vi "RX-SIM-BPCS-UDP.vi"() -> ()   [LabVIEW 2018]
uses:
  <vilib>/Platform/TimedLoop/XDataNode/timing_clust.ctl
  <vilib>/Platform/TimedLoop/XDataNode/nitl_modes.ctl
  <vilib>/Platform/TimedLoop/XDataNode/wakeup.ctl
  Modbus/ControllersHost/BPCS Global Variables.vi
  <vilib>/Platform/TimedLoop/XDataNode/XDataNode.xnode
  <vilib>/Platform/TimedLoop/XDataNode/XDNodeRunTimeDep.lvlib
panel:
  in  "Stop":bool
  out "SIM-BPCS-RX-ARRAY":dbl[](array[numeric])
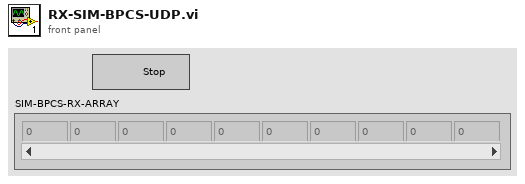
[diagram p1: front panel]
types:
  T1 = typedef "XDNodeRunTimeDep.lvlib/timing_clust.ctl" = cluster{"Expected End [f-1]":u64, "Actual End [f-1]":u64, "Finished Late? [f-1]":bool, "Expected End [i-1]":u64, "Actual End [i-1]":u64, "Finished Late? [i-1]":bool, "Expected Start [i]":u64, "Actual Start [i]":u64, "Expected Start [f]":u64, "Actual Start [f]":u64, "Source Name":string, "Structure Name":string, "Period":i64, "Deadline":i64, "Offset":i64, "Start":i64, "Priority":i32, "Timeout":i32, "Mode":T2, "Wakeup Reason":T3, "Error":errorcluster, "Source Type":string, "Secondary Source Type":string, "Global End Time":u64, "Global Start Time":u64, "Frame Duration":u64, "Iteration Duration":u64, "Assigned CPU":i32, "I/O Scan Engine Mode":u32}
  T2 = typedef "XDNodeRunTimeDep.lvlib/nitl_modes.ctl" = enum32{"No Change", "Process missed periods, maintain original phase", "Discard missed periods, maintain original phase", "Process missed periods, ignore original phase", "Discard missed periods, ignore original phase"}
  T3 = typedef "XDNodeRunTimeDep.lvlib/wakeup.ctl" = enum32{"Normal", "Aborted", "Asynchronous wakeup", "Timing source error", "Timed loop error", "Timeout"}
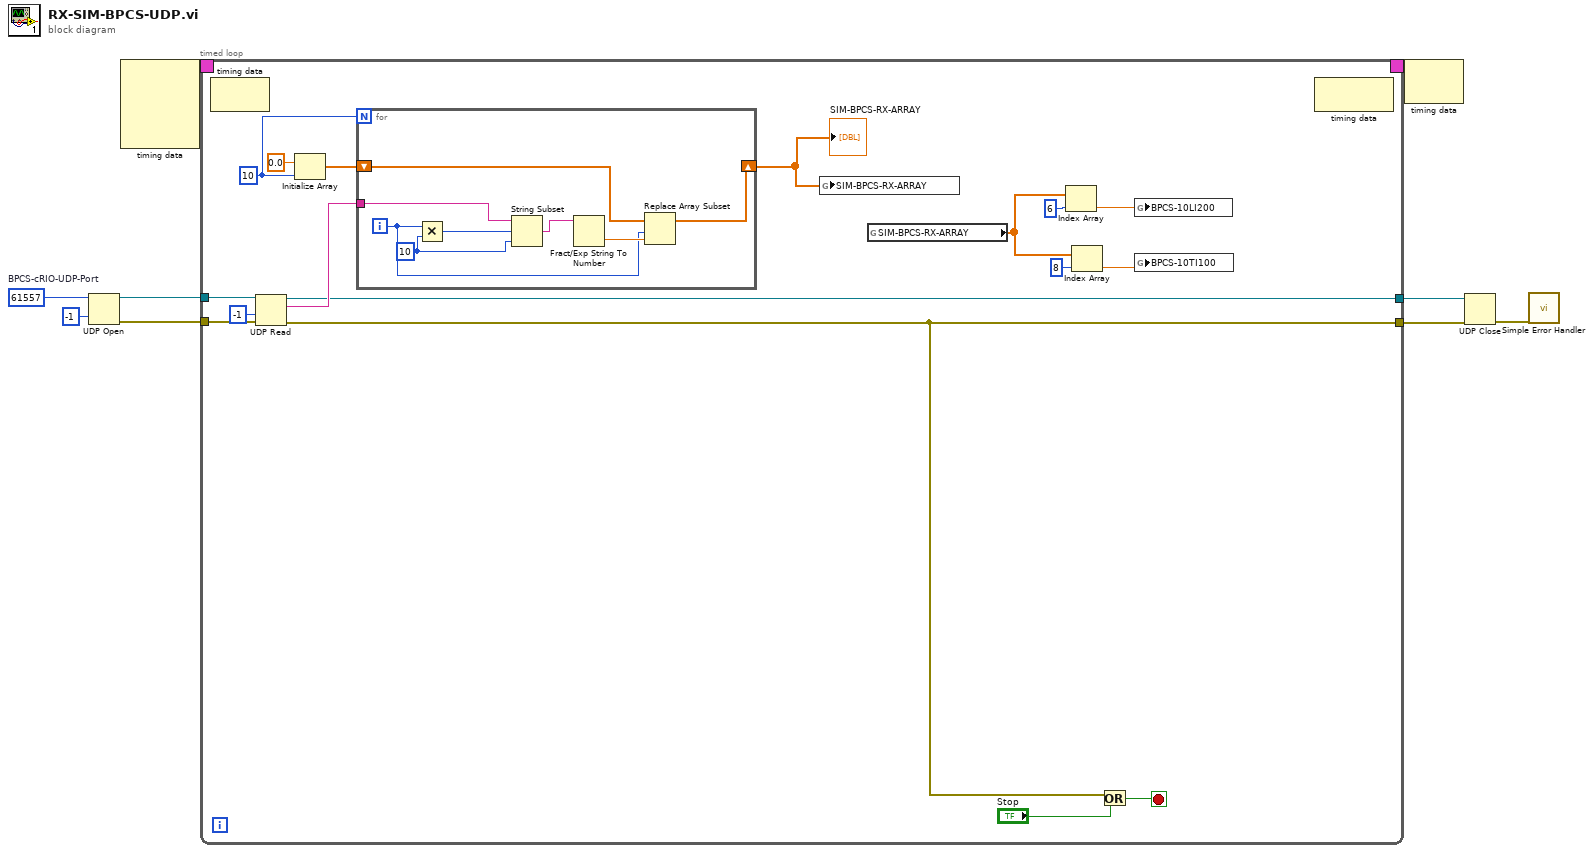
[diagram p0: block diagram]
diagram:
  w7 = u16 61557  # BPCS-cRIO-UDP-Port
  n1 = UDP Open(9:-1 ("timeout ms (25000)"), 11:w7) -> (port=w6:refnum<k16>, 0:w5:errorcluster)  [unwired: 3 in, 1 out]
  n2 = node-c288() -> (w9:T1)  [unwired: 4 in]
  n3 = timed-loop {
    timing: w9 -> [_]
    timing-out: [_] -> w8
    tunnel: w6 -> [w24]
    tunnel: w5 -> [w23]
    tunnel: [w21] -> w3
    tunnel: [w15] -> w1
    stop <- w25 stop-if-true
    w18 = 10 ("dimension size")
    n4 = node-c288() -> ()  [unwired: 1 in, 1 out]
    n5 = UDP Read(connection ID=w24, timeout ms (25000)=-1, 8:w23) -> (data out=w22:string, error out=w15:errorcluster, 3:w21:refnum<k16>)  [unwired: 3 out]
    n6 = Initialize Array(0.0 ("element"), w18) -> (w19:dbl[])
    n7 = for {
      N: w18 -> [_]
      tunnel: w22 -> [w33]
      shift-right: [w29] -> w16
      shift-left: w19 -> [w28]
      i -> [w30]
      w27 = 10 ("y")
      n8 = Multiply(x=w30, y=w27) -> (x*y=w32:i32)
      n9 = String Subset(string=w33, offset (0)=w32, length (rest)=w27) -> (substring=w34:string)
      n10 = Fract/Exp String To Number(string=w34) -> (number=w31:dbl)  [unwired: 3 in, 1 out]
      n11 = Replace Array Subset(array=w28, new element=w31, index=w30) -> (w29:dbl[])
    }
    "SIM-BPCS-RX-ARRAY" <- w16
    n12 = global write "BPCS Global Variables.vi" "SIM-BPCS-RX-ARRAY"(w16) -> ()
    n13 = global read "BPCS Global Variables.vi" "SIM-BPCS-RX-ARRAY"() -> (w12:dbl[])
    n14 = Index Array(array=w12, index=6) -> (element=w11:dbl)
    n15 = Index Array(array=w12, index=8) -> (element=w10:dbl)
    n16 = Or(x=w15, y="Stop") -> (x .or. y?=w25:bool)
    n17 = global write "BPCS Global Variables.vi" "BPCS-10LI200"(w11) -> ()
    n18 = global write "BPCS Global Variables.vi" "BPCS-10TI100"(w10) -> ()
    n19 = node-c288() -> ()  [unwired: 1 in, 1 out]
  }
  n20 = node-c288(w8) -> ()  [unwired: 1 out]
  n21 = UDP Close(connection ID=w3, 8:w1) -> (error out=w4:errorcluster)  [unwired: 1 out]
  n22 = call <vilib>:"Simple Error Handler.vi"("error in (no error)"=w4) -> ()  [unwired: 4 in, 5 out]
